vi "校准任务设置.vi"(8 "校准触发任务":refnum<user-event>, 9 "精度":dbl=4.0, 10 "模型":enum32{"线性", "多项式"}(ring), 11 "用户事件":refnum<user-event>) -> ()   [LabVIEW 2016, in "斯坦道总磷.lvlib"]
uses:
  <vilib>/Utility/xml.llb/Write to XML File(string).vi
  <vilib>/Utility/xml.llb/Read From XML File(string).vi
panel:
  out "参数":u16
  in  "导入":bool
  in  "保存":bool
  in  "校准任务存档":T1[](array[typedef])
  out "字符串":string
  out "校准运行状态":bool
  in  "校准任务":T1[](array[typedef])
  in  "停止":bool
  in  "设置":bool
  in  "执行":bool
  in  "删除":bool
  in  "清空":bool
  in  "任务列表":i32(listbox)
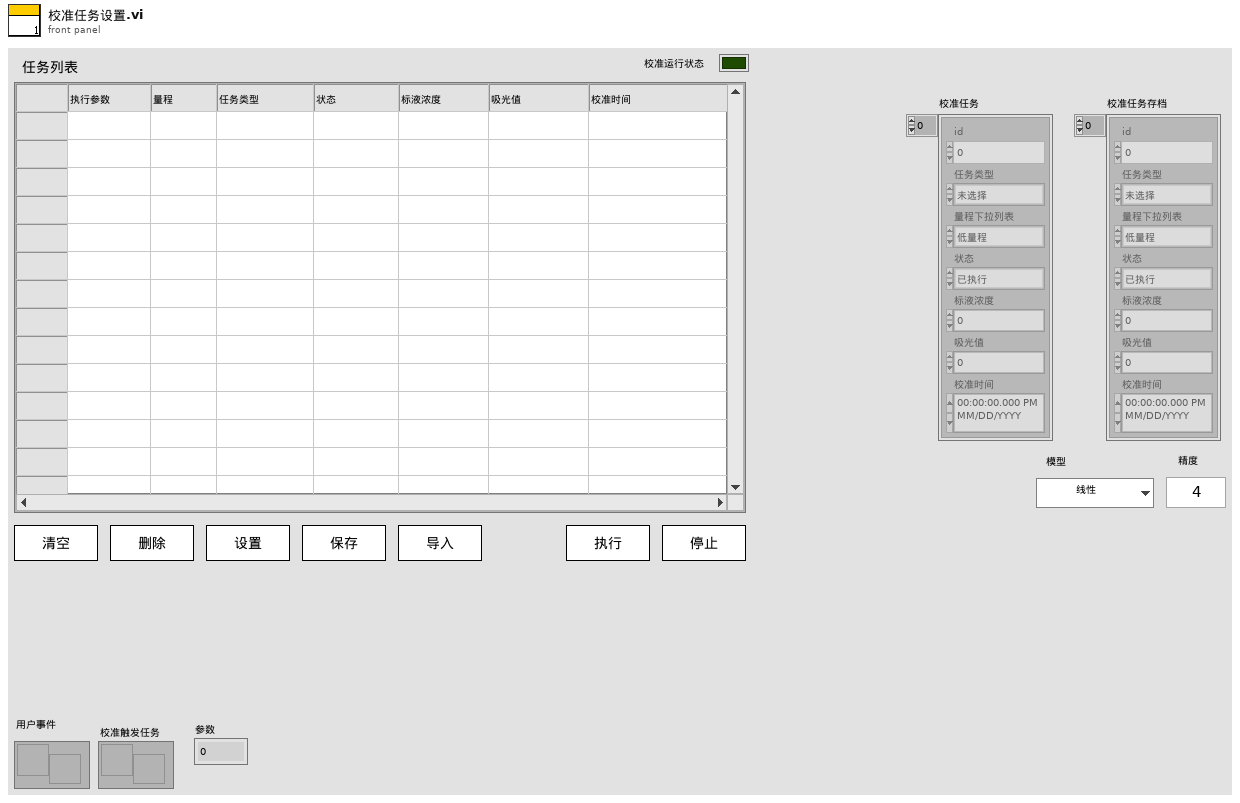
[diagram p1: front panel]
types:
  T1 = typedef "斯坦道总磷.lvlib/校准任务.ctl" = cluster{"id":u16, "任务类型":enum16{"未选择", "空白校准", "标样校准", "标样核查", "零点核查", "跨度核查"}, "量程下拉列表":enum16{"低量程", "高量程"}, "状态":enum16{"已执行", "待执行", "执行中", "停止"}, "标液浓度":dbl, "吸光值":dbl, "校准时间":timestamp}
  T2 = cluster{"校准类型":string, "校准数据":cluster{"时间":timestamp, "标液值":dbl, "检测值":dbl, "吸光值":dbl}}
  T3 = enum8{"Enabled", "Disabled", "Disabled and Grayed Out"}
  T4 = typedef "斯坦道总磷总氮.lvlib/校准任务.ctl" = cluster{"id":u16, "任务类型":enum16{"未选择", "空白校准", "标样校准", "标样核查", "零点核查", "跨度核查"}, "量程下拉列表":enum16{"低量程", "高量程"}, "状态":enum16{"已执行", "待执行", "执行中", "停止"}, "标液浓度":dbl, "吸光值":dbl, "校准时间":timestamp}
  T5 = typedef "LVPoint32TypeDef.ctl" = cluster{"Horizontal":i32, "Vertical":i32}
  T6 = typedef "LVRowAndColumnTypeDef.ctl" = cluster{"Row":i32, "Column":i32}
  T7 = enum16{"未选择", "空白校准", "标样校准", "标样核查", "零点核查", "跨度核查"}
  T8 = cluster{"id":u16, "任务类型":enum16{"未选择", "空白校准", "标样校准", "标样核查", "零点核查", "跨度核查"}, "量程下拉列表":enum16{"低量程", "高量程"}, "状态":enum16{"已执行", "待执行", "执行中", "停止"}, "标液浓度":dbl, "吸光值":dbl, "校准时间":timestamp}
  T9 = enum32{"Bad", "Idle", "Run top level", "Running"}
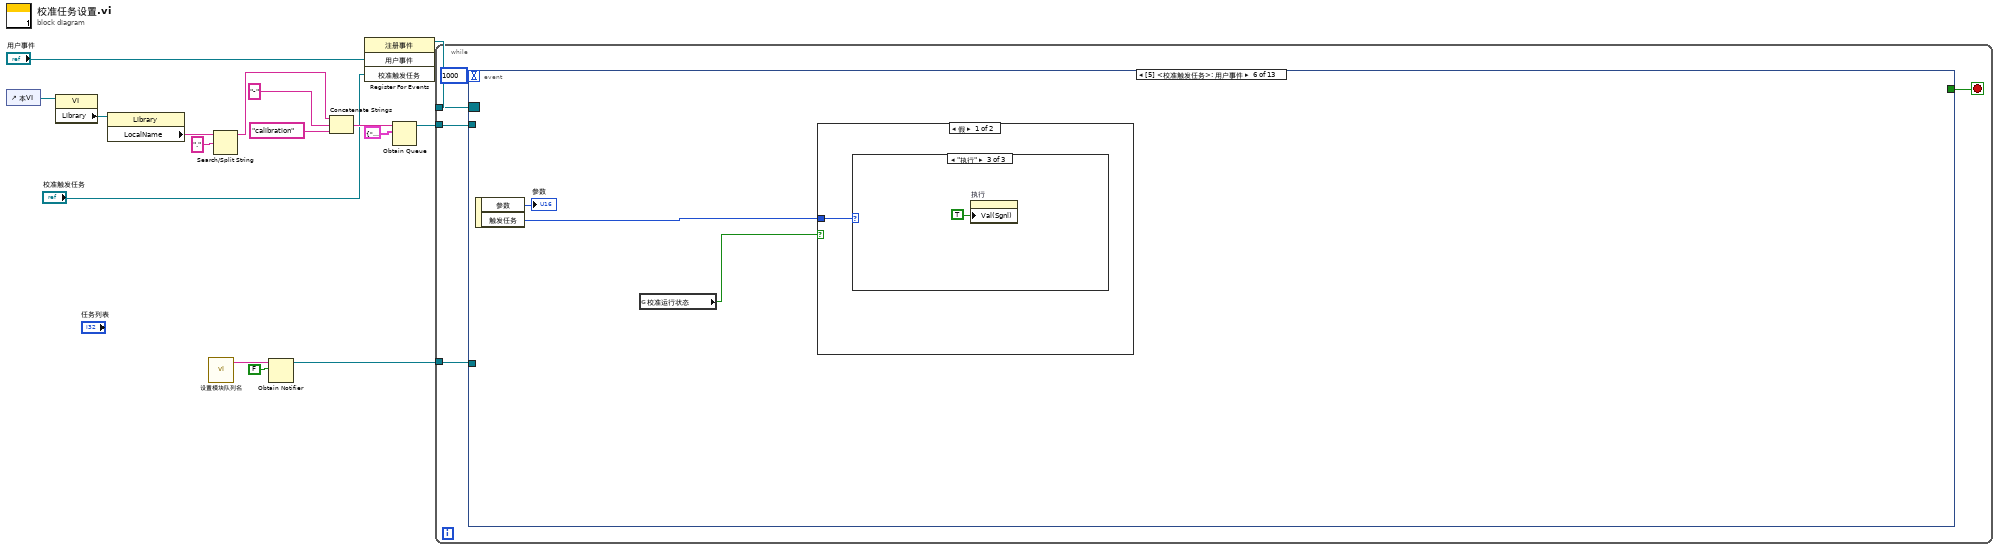
[diagram p0: block diagram]
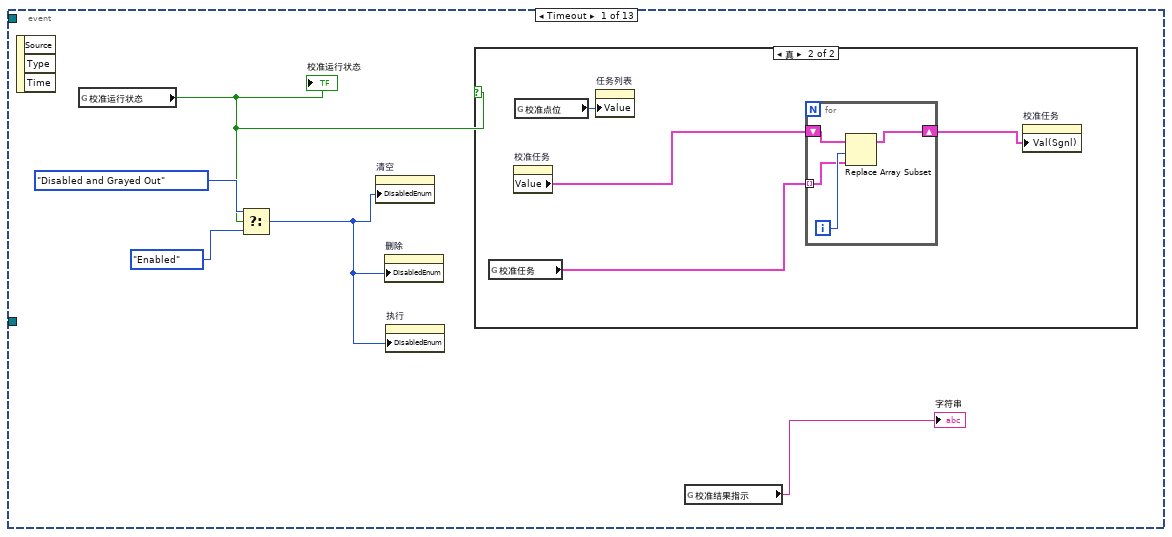
[diagram p2: hidden frame]
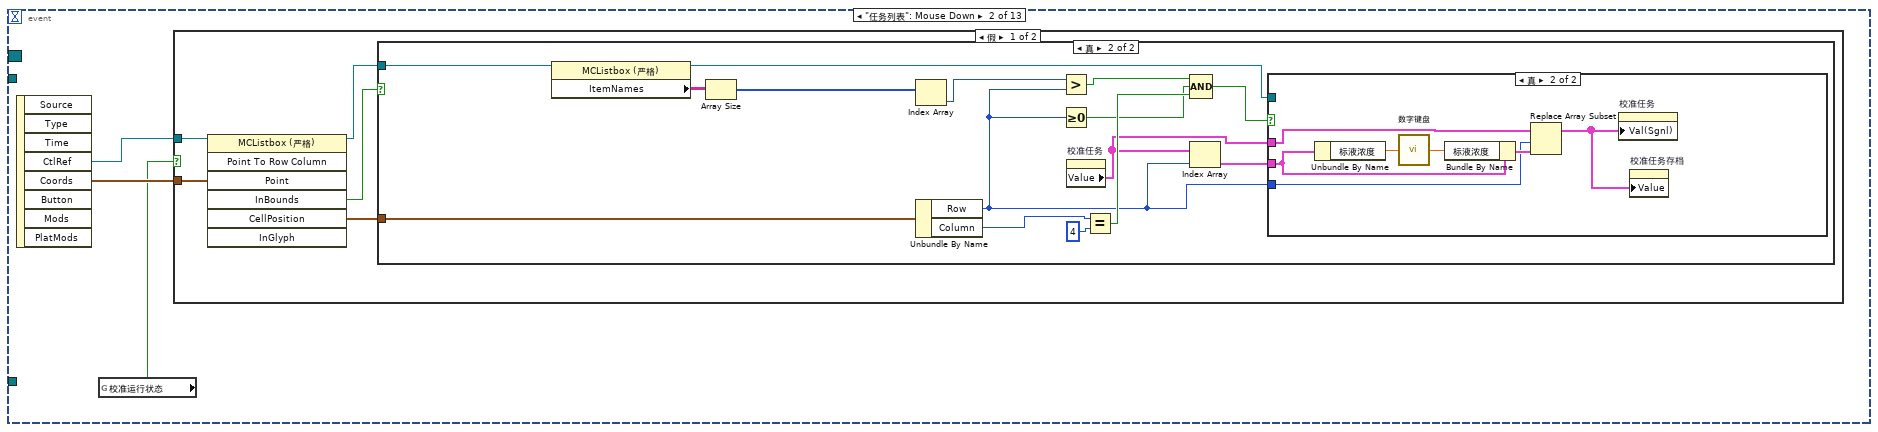
[diagram p4: hidden frame]
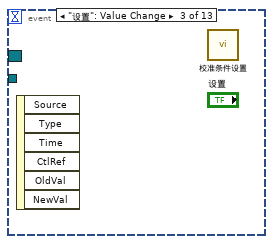
[diagram p8: hidden frame]
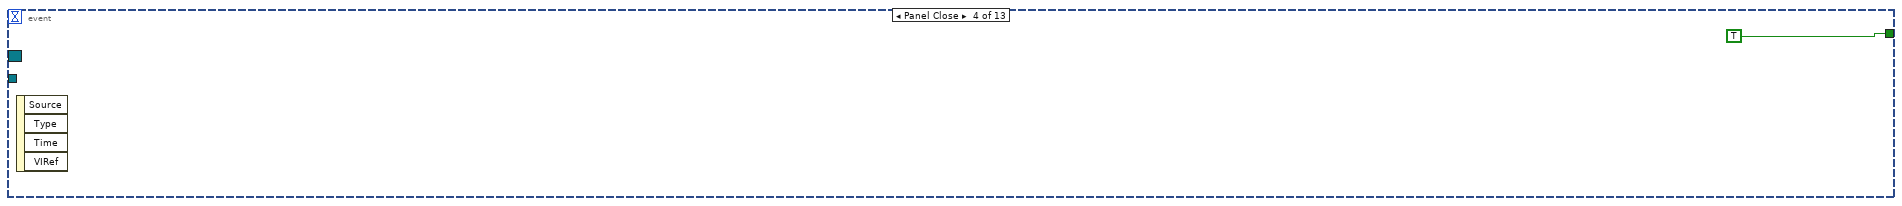
[diagram p9: hidden frame]
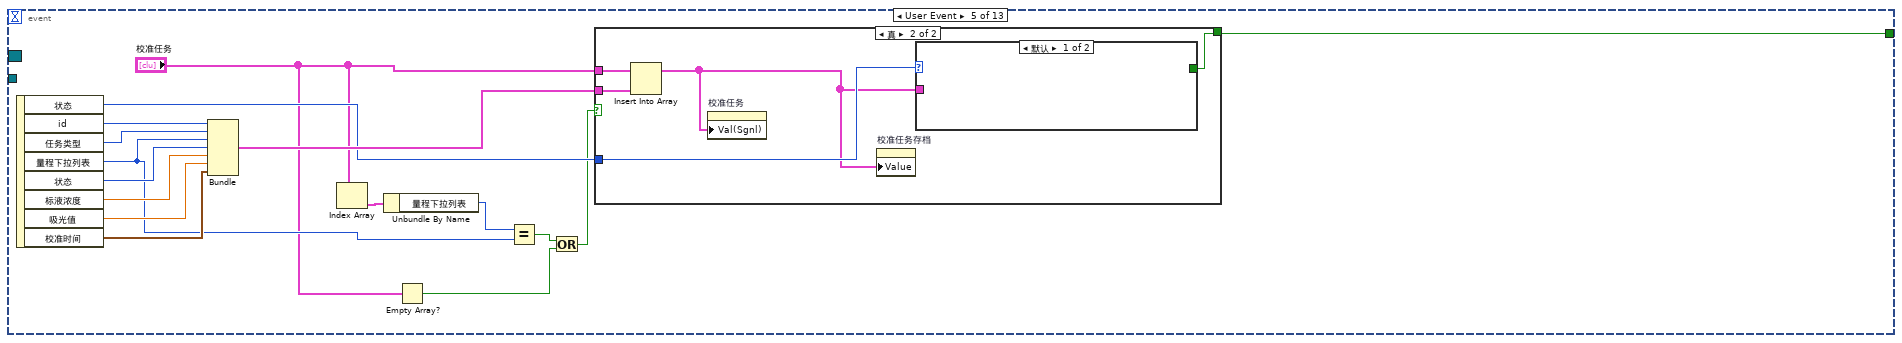
[diagram p10: hidden frame]
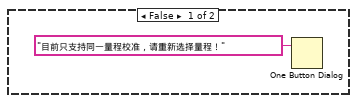
[diagram p11: hidden frame]
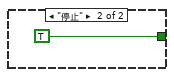
[diagram p12: hidden frame]
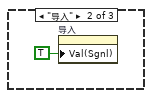
[diagram p14: hidden frame]
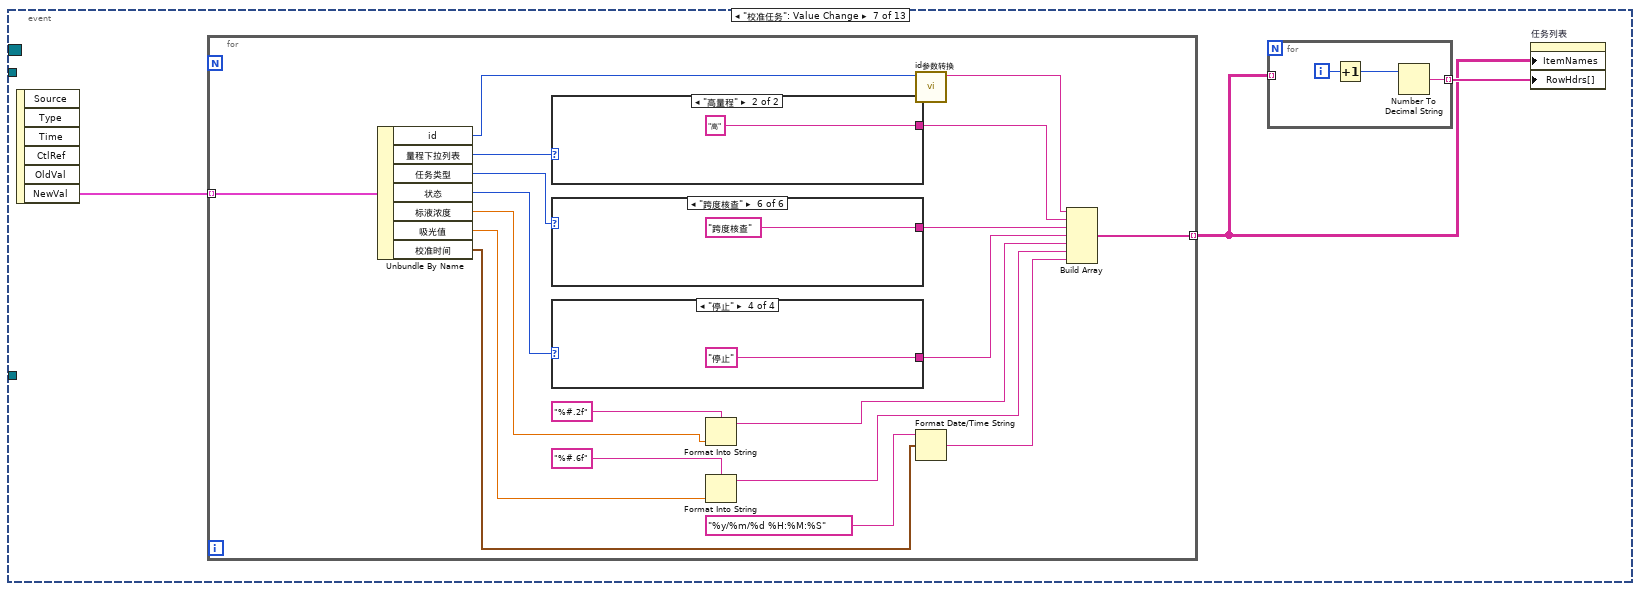
[diagram p16: hidden frame]
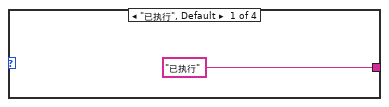
[diagram p17: hidden frame]
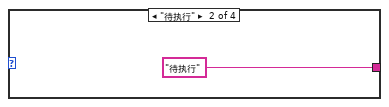
[diagram p18: hidden frame]
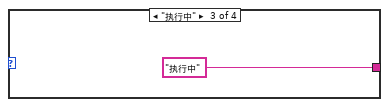
[diagram p19: hidden frame]
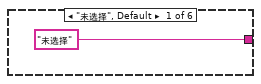
[diagram p20: hidden frame]
diagram:
  n1 = control-ref of="本VI"() -> (w15:refnum<vi>)
  n2 = property class="VI"(reference=w15) -> ("Library"=w16:refnum<vi>)  [unwired: 1 in, 2 out]
  n3 = property class="Library"(reference=w16) -> ("LocalName"=w14:string)  [unwired: 1 in, 2 out]
  n4 = call "设置模块队列名.vi"() -> ("Msg"=w3:string)  [unwired: 5 in]
  n5 = Search/Split String(string=w14, search string/char (-)="." ("搜索字符串/字符(-)")) -> (substring before match=w12:string)  [unwired: 1 in, 2 out]
  n6 = Obtain Notifier(name (unnamed)=w3, notification data type=FALSE) -> (notifier out=w2:refnum<notifier>)  [unwired: 2 in, 2 out]
  n7 = Concatenate Strings(w12, "-" ("字符串"), "calibration" ("名称或相对路径")) -> (w9:string)
  n8 = register-events("用户事件", "校准触发任务") -> (reference out=w6:refnum<event-registration>)  [unwired: 2 in, 1 out]
  n9 = Obtain Queue(name (unnamed)=w9, element data type=T2 {"校准类型"="", "校准数据"={"时间"=timestamp(0 s since 1904-01-01), "标液值"=0.0, "检测值"=0.0, "吸光值"=0.0}}) -> (queue out=w7:refnum<queue>)  [unwired: 3 in, 2 out]
  n10 = while {
    tunnel: w7 -> [w20]
    tunnel: w6 -> [w19]
    tunnel: w2 -> [w18]
    stop <- w21 stop-if-true
    n11 = event shown="[5] <校准触发任务>: 用户事件" {
      selector: w19 -> [_ _ _ _ _ _ _ _ _ _ _ _ _]
      dyn-events: _ -> [_ _ _ _ _ _ _ _ _ _ _ _ _]
      timeout: 1000 -> [_ _ _ _ _ _ _ _ _ _ _ _ _]
      tunnel: [_ _ _ TRUE w81 _ _ _ _ _ _ _ _] -> w21
      tunnel: w20 -> [_ _ _ _ _ _ _ _ _ _ _ _ _]
      tunnel: w18 -> [_ _ _ _ _ _ _ _ _ _ w154 _ _]
      event Timeout {
        n12 = event-data() -> ()  [unwired: 1 in, 3 out]
        n13 = global read "VAR总磷总氮全局变量.vi" "校准运行状态"() -> (w23:bool)
        "校准运行状态" <- w23
        n14 = Select(t=T3."Disabled and Grayed Out" ("禁用"), s=w23, f=T3."Enabled" ("禁用")) -> (s? t:f=w25:T3)
        n15 = property on="清空" class="Bool"("DisabledEnum"=w25) -> ()  [unwired: 2 in, 2 out]
        n16 = property on="删除" class="Bool"("DisabledEnum"=w25) -> ()  [unwired: 2 in, 2 out]
        n17 = property on="执行" class="Bool (严格)"("DisabledEnum"=w25) -> ()  [unwired: 2 in, 2 out]
        n18 = case shown="真" w23 {
          frame False {
          }
          frame True {
            n19 = global read "VAR总磷总氮全局变量.vi" "校准任务"() -> (w28:T1[])
            n20 = property on="校准任务" class="Arr (严格)"() -> ("Value"=w29:T4[])  [unwired: 2 in, 2 out]
            n21 = global read "VAR总磷总氮全局变量.vi" "校准点位"() -> (w30:u16)
            n22 = property on="任务列表" class="MCListbox (严格)"("Value"=w30) -> ()  [unwired: 2 in, 2 out]
            n23 = for {
              tunnel: w28 -> [w32] mode=indexing
              shift-right: [w31] -> w27
              shift-left: w29 -> [w34]
              i -> [w33]
              n24 = Replace Array Subset(array=w34, new element=w32, index=w33) -> (w31:T4[])
            }
            n25 = property on="校准任务" class="Arr (严格)"("Val(Sgnl)"=w27) -> ()  [unwired: 2 in, 2 out]
          }
        }
        n26 = global read "VAR总磷总氮全局变量.vi" "校准结果指示"() -> (→"字符串":string)
      }
      event "任务列表": Mouse Down {
        n27 = event-data() -> ("CtlRef"=w37:refnum<vi>, "Coords"=w36:T5)  [unwired: 1 in, 6 out]
        n28 = global read "VAR总磷总氮全局变量.vi" "校准运行状态"() -> (w35:bool)
        n29 = case shown="假" w35 {
          tunnel: w37 -> [w42 _]
          tunnel: w36 -> [w38 _]
          frame False {
            n30 = invoke class="MCListbox (严格)" method="Point To Row Column"(reference=w42, "Point"=w38) -> (reference out=w39:refnum<vi>, "InBounds"=w41:bool, "CellPosition"=w40:T6)  [unwired: 5 in, 4 out]
            n31 = case shown="真" w41 {
              tunnel: w40 -> [_ w57]
              tunnel: w39 -> [_ w56]
              frame False {
              }
              frame True {
                n32 = property class="MCListbox (严格)"(reference=w56) -> (reference out=w55:refnum<vi>, "ItemNames"=w54:string[][])  [unwired: 1 in, 1 out]
                n33 = Array Size(array=w54) -> (size(s)=w53:i32[])
                n34 = Index Array(array=w53) -> (element=w52:i32)  [unwired: 1 in]
                n35 = Unbundle By Name(w57) -> ("Row"=w43:i32, "Column"=w51:i32)
                n36 = Greater?(x=w52, y=w43) -> (0:w47:bool)
                n37 = Greater Or Equal To 0?(x=w43) -> (x >= 0?=w46:bool)
                n38 = property on="校准任务" class="Arr (严格)"() -> ("Value"=w44:T4[])  [unwired: 2 in, 2 out]
                n39 = Equal?(x=w51, y=4) -> (x = y?=w49:bool)
                n40 = Compound Arithmetic op=AND ("复合运算")(w47, w46, w49) -> (w48:bool)
                n41 = Index Array(array=w44, index=w43) -> (element=w45:T4)
                n42 = case shown="真" w48 {
                  tunnel: w55 -> [_ _]
                  tunnel: w45 -> [_ w63]
                  tunnel: w44 -> [_ w61]
                  tunnel: w43 -> [_ w59]
                  frame False {
                  }
                  frame True {
                    n43 = Unbundle By Name(w63) -> ("标液浓度"=w64:dbl)
                    n44 = call "数字键盘.vi"("OldNumber"=w64) -> ("NewNumber"=w62:dbl)
                    n45 = Bundle By Name(cluster=w63, "标液浓度"=w62) -> (w60:T4)
                    n46 = Replace Array Subset(array=w61, new element=w60, index=w59) -> (w58:T4[])
                    n47 = property on="校准任务" class="Arr (严格)"("Val(Sgnl)"=w58) -> ()  [unwired: 2 in, 2 out]
                    n48 = property on="校准任务存档" class="Arr (严格)"("Value"=w58) -> ()  [unwired: 2 in, 2 out]
                  }
                }
              }
            }
          }
          frame True {
          }
        }
      }
      event "设置": Value Change {
        n49 = event-data() -> ()  [unwired: 1 in, 6 out]
        n50 = call "校准条件设置.vi"() -> ()  [unwired: 12 in]
      }
      event Panel Close {
        n51 = event-data() -> ()  [unwired: 1 in, 4 out]
      }
      event User Event {
        n52 = event-data() -> ("状态"=w73:enum16{"已执行", "待执行", "执行中", "停止"}, "id"=w80:u16, "任务类型"=w78:T7, "量程下拉列表"=w70:enum16{"低量程", "高量程"}, "状态"=w77:enum16{"已执行", "待执行", "执行中", "停止"}, "标液浓度"=w76:dbl, "吸光值"=w75:dbl, "校准时间"=w74:timestamp)  [unwired: 1 in]
        n53 = Bundle("id"=w80, "任务类型"=w78, "量程下拉列表"=w70, "状态"=w77, "标液浓度"=w76, "吸光值"=w75, "校准时间"=w74) -> (w79:T8)  [unwired: 1 in]
        n54 = Index Array(array="校准任务") -> (element=w72:T1)  [unwired: 1 in]
        n55 = Unbundle By Name(w72) -> ("量程下拉列表"=w71:enum16{"低量程", "高量程"})
        n56 = Empty Array?(array="校准任务") -> (empty?=w66:bool)
        n57 = Equal?(x=w71, y=w70) -> (x = y?=w68:bool)
        n58 = Or(x=w68, y=w66) -> (x .or. y?=w67:bool)
        n59 = case shown="真" w67 {
          tunnel: [_ w87] -> w81
          tunnel: w79 -> [_ w86]
          tunnel: w73 -> [_ w85]
          tunnel: "校准任务" -> [_ w84]
          frame False {
            n60 = One Button Dialog(message="目前只支持同一量程校准，请重新选择量程！" ("消息")) -> ()  [unwired: 1 in, 1 out]
          }
          frame True {
            n61 = Insert Into Array(array=w84, new element=w86) -> (w83:T1[])  [unwired: 1 in]
            n62 = property on="校准任务" class="Arr (严格)"("Val(Sgnl)"=w83) -> ()  [unwired: 2 in, 2 out]
            n63 = property on="校准任务存档" class="Arr (严格)"("Value"=w83) -> ()  [unwired: 2 in, 2 out]
            n64 = case shown="默认" w85 {
              tunnel: [_ TRUE] -> w87
              tunnel: w83 -> [_ _]
              frame Default {
              }
              frame "停止" {
              }
            }
          }
        }
      }
      event User Event {
        n65 = event-data() -> ("参数"=→"参数":u16, "触发任务"=w91:enum16{"Non", "导入", "执行"})  [unwired: 1 in]
        n66 = global read "VAR总磷总氮全局变量.vi" "校准运行状态"() -> (w89:bool)
        n67 = case shown="假" w89 {
          tunnel: w91 -> [w92 _]
          frame False {
            n68 = case shown="\"执行\"" w92 {
              frame "Non", Default {
              }
              frame "导入" {
                n69 = property on="导入" class="Bool (严格)"("Val(Sgnl)"=TRUE ("值(信号)")) -> ()  [unwired: 2 in, 2 out]
              }
              frame "执行" {
                n70 = property on="执行" class="Bool (严格)"("Val(Sgnl)"=TRUE ("值(信号)")) -> ()  [unwired: 2 in, 2 out]
              }
            }
          }
          frame True {
          }
        }
      }
      event "校准任务": Value Change {
        n71 = event-data() -> ("NewVal"=w95:T1[])  [unwired: 1 in, 5 out]
        n72 = for {
          tunnel: w95 -> [w116] mode=indexing
          tunnel: [w98] -> w96 mode=indexing
          n73 = Unbundle By Name(w116) -> ("id"=w115:u16, "量程下拉列表"=w114:enum16{"低量程", "高量程"}, "任务类型"=w113:T7, "状态"=w112:enum16{"已执行", "待执行", "执行中", "停止"}, "标液浓度"=w110:dbl, "吸光值"=w108:dbl, "校准时间"=w106:timestamp)
          n74 = case shown="\"高量程\"" w114 {
            tunnel: ["低" "高"] -> w104
            frame "低量程", Default {
            }
            frame "高量程" {
            }
          }
          n75 = case shown="\"跨度核查\"" w113 {
            tunnel: ["未选择" "空白校准" "标样校准" "标样核查" "零点核查" "跨度核查"] -> w103
            frame "未选择", Default {
            }
            frame "空白校准" {
            }
            frame "标样校准" {
            }
            frame "标样核查" {
            }
            frame "零点核查" {
            }
            frame "跨度核查" {
            }
          }
          n76 = case shown="\"停止\"" w112 {
            tunnel: ["已执行" "待执行" "执行中" "停止"] -> w102
            frame "已执行", Default {
            }
            frame "待执行" {
            }
            frame "执行中" {
            }
            frame "停止" {
            }
          }
          n77 = Format Into String(format string="%#.2f" ("格式字符串"), w110) -> (resulting string=w101:string)  [unwired: 2 in, 1 out]
          n78 = Format Into String(format string="%#.6f" ("格式字符串"), w108) -> (resulting string=w100:string)  [unwired: 2 in, 1 out]
          n79 = call "id参数转换.vi"("id"=w115) -> ("table输出"=w105:string)  [unwired: 9 in, 1 out]
          n80 = Format Date/Time String(time format string (%c)="%y/%m/%d %H:%M:%S" ("时间格式字符串(%c)"), seconds (now)=w106) -> (date/time string=w99:string)  [unwired: 1 in]
          n81 = Build Array(w105, w104, w103, w102, w101, w100, w99) -> (w98:string[])
        }
        n82 = for {
          tunnel: [w129] -> w97 mode=indexing
          tunnel: w96 -> [_] mode=indexing
          i -> [w131]
          n83 = Increment(x=w131) -> (x+1=w130:i32)
          n84 = Number To Decimal String(number=w130) -> (decimal integer string=w129:string)  [unwired: 1 in]
        }
        n85 = property on="任务列表" class="MCListbox (严格)"("ItemNames"=w96, "RowHdrs[]"=w97) -> ()  [unwired: 2 in, 2 out]
      }
      event "清空": Value Change {
        n86 = event-data() -> ()  [unwired: 1 in, 6 out]
        n87 = property on="校准任务" class="Arr (严格)"("Val(Sgnl)"=T1[] [] ("数组")) -> ()  [unwired: 2 in, 2 out]
      }
      event "删除": Value Change {
        n88 = event-data() -> ()  [unwired: 1 in, 6 out]
        n89 = property on="校准任务" class="Arr (严格)"() -> ("Value"=w135:T4[])  [unwired: 2 in, 2 out]
        n90 = property on="任务列表" class="MCListbox (严格)"() -> ("Value"=w133:i32)  [unwired: 2 in, 2 out]
        n91 = Delete From Array(array=w135, index=w133) -> (array with subset deleted=w134:T4[])  [unwired: 1 in, 1 out]
        n92 = property on="校准任务" class="Arr (严格)"("Val(Sgnl)"=w134) -> ()  [unwired: 2 in, 2 out]
      }
      event "执行": Value Change {
        n93 = event-data() -> ()  [unwired: 1 in, 6 out]
        n94 = local write "执行"(FALSE ("执行")) -> ()
        n95 = vi-ref "校准任务流程.vi"() -> (w138:refnum<vi>)
        n96 = property class="VI"(reference=w138) -> (reference out=w141:refnum<vi>, "Name"=w139:string, "Exec.State"=w140:T9)  [unwired: 1 in, 1 out]
        n97 = case shown="\"Idle\"" w140 {
          tunnel: w139 -> [_ w152]
          tunnel: w141 -> [_ _]
          tunnel: "模型" -> [_ w145]
          tunnel: "精度" -> [_ w144]
          frame "Bad", Default {
          }
          frame "Idle" {
            n98 = Open VI Reference(type specifier VI Refnum (for type only)=refnum<vi> refnum, vi path=w152, options=128 ("选项")) -> (vi reference=w150:refnum<vi>, error out=w148:errorcluster)  [unwired: 3 in]
            n99 = call-by-ref "开始异步调用"(reference=w150, error in=w148, "校准任务"="校准任务存档", "精度"=w144, "模型"=w145) -> (reference out=w149:refnum<vi>, error out=w147:errorcluster)  [unwired: 9 in]
            n100 = Close Reference(reference=w149, error in (no error)=w147) -> ()  [unwired: 1 out]
          }
        }
      }
      event "停止": Value Change {
        n101 = event-data() -> ()  [unwired: 1 in, 6 out]
        n102 = Send Notification(notification=TRUE ("通知"), notifier=w154) -> ()  [unwired: 1 in, 2 out]
      }
      event "保存": Value Change {
        n103 = event-data() -> ()  [unwired: 1 in, 6 out]
        n104 = property on="校准任务" class="Arr (严格)"() -> ("Value"=w156:T4[])  [unwired: 2 in, 2 out]
        n105 = for {
          tunnel: w156 -> [w171] mode=indexing
          tunnel: [w170] -> w159 mode=indexing
          n106 = in-place {
            n107 = in-place-cluster #1(w171) -> ()  [unwired: 1 out]
            n108 = in-place-cluster #1("状态"=enum16{"已执行", "待执行", "执行中", "停止"}."待执行") -> (w170:T4)
          }
        }
        n109 = control-ref of="本VI"() -> (w165:refnum<vi>)
        n110 = property class="VI"(reference=w165) -> ("Library"=w166:refnum<vi>)  [unwired: 1 in, 2 out]
        n111 = local write "保存"(FALSE ("保存")) -> ()
        n112 = property class="Library"(reference=w166) -> ("LocalName"=w163:string)  [unwired: 1 in, 2 out]
        n113 = call <vilib>:"Application Directory.vi"() -> ("Application Directory"=w169:path)
        n114 = Search/Split String(string=w163, search string/char (-)="." ("搜索字符串/字符(-)")) -> (substring before match=w162:string)  [unwired: 1 in, 2 out]
        n115 = Build Path(base path=w169, name or relative path="config" ("名称或相对路径")) -> (appended path=w167:path)
        n116 = Concatenate Strings(w162, "CalTask.xml" ("字符串")) -> (w161:string)
        n117 = Build Path(base path=w167, name or relative path=w161) -> (appended path=w157:path)
        n118 = Flatten To XML(anything=w159) -> (xml string=w158:string)
        n119 = call-poly <vilib>:"Write to XML File.vi"("XML Input"=w158, "XML File Path"=w157) -> ()  [unwired: 7 in, 3 out]
      }
      event "导入": Value Change {
        n120 = event-data() -> ()  [unwired: 1 in, 6 out]
        n121 = local write "导入"(FALSE ("导入")) -> ()
        n122 = control-ref of="本VI"() -> (w184:refnum<vi>)
        n123 = property class="VI"(reference=w184) -> ("Library"=w185:refnum<vi>)  [unwired: 1 in, 2 out]
        n124 = property class="Library"(reference=w185) -> ("LocalName"=w182:string)  [unwired: 1 in, 2 out]
        n125 = call <vilib>:"Application Directory.vi"() -> ("Application Directory"=w188:path)
        n126 = Search/Split String(string=w182, search string/char (-)="." ("搜索字符串/字符(-)")) -> (substring before match=w181:string)  [unwired: 1 in, 2 out]
        n127 = Build Path(base path=w188, name or relative path="config" ("名称或相对路径")) -> (appended path=w186:path)
        n128 = Concatenate Strings(w181, "CalTask.xml" ("字符串")) -> (w180:string)
        n129 = Build Path(base path=w186, name or relative path=w180) -> (appended path=w178:path)
        n130 = call-poly <vilib>:"Read From XML File.vi"("XML File Path"=w178) -> ("XML Elements"=w177:string)  [unwired: 8 in, 2 out]
        n131 = local read "校准任务"() -> (w176:T1[])
        n132 = Unflatten From XML(xml string=w177, type=w176) -> (value=w174:T1[])  [unwired: 1 in, 1 out]
        n133 = for {
          tunnel: w174 -> [w190] mode=indexing
          tunnel: [w190] -> w173 mode=indexing if=w189
          n134 = local read "参数"() -> (w191:u16)
          n135 = Unbundle By Name(w190) -> ("id"=w192:u16)
          n136 = Equal?(x=w192, y=w191) -> (x = y?=w189:bool)
        }
        n137 = local write "校准任务存档"(w173) -> ()
        n138 = property on="校准任务" class="Arr (严格)"("Val(Sgnl)"=w173) -> ()  [unwired: 2 in, 2 out]
      }
    }
  }
